vi "getMessage.vi"(8 "error in (no error)":errorcluster, 9 "mode (standard)":T1(ring)=enum."CRLF", 10 "bytes to read":i32=2048, 11 "TCPClient in":refnum<class "TCPClient.lvclass">) -> (0 "error out":errorcluster, 2 "message":string, 3 "TCPClient out":refnum<class "TCPClient.lvclass">)   [LabVIEW 2016, in "tcp.lvlib" / "TCPClient.lvclass"]
uses:
  TCPClient.lvclass
  TCPClient.lvclass/TCPClient.ctl
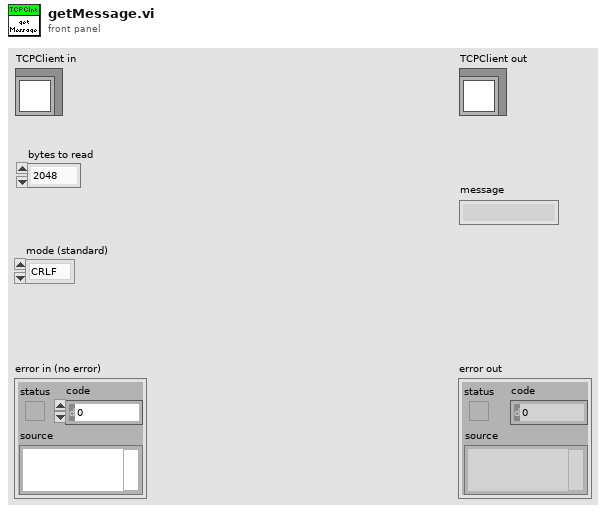
[diagram p1: front panel]
types:
  T1 = enum16{"Standard", "Buffered", "CRLF", "Immediate"}
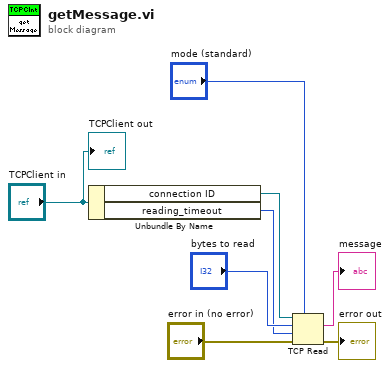
[diagram p0: block diagram]
diagram:
  n1 = Unbundle By Name("TCPClient in") -> ("connection ID"=w1:refnum<k5>, "reading_timeout"=w2:i32)
  n2 = TCP Read(connection ID=w1, bytes to read="bytes to read", error in (no error)="error in (no error)", 7:"mode (standard)", 9:w2) -> (data out=→"message":string, error out=→"error out":errorcluster)  [unwired: 1 out]
  "TCPClient out" <- "TCPClient in"
